vi "Index Event in Device List.vi"(8 "Error In":errorcluster, 11 "Device List State":T1) -> (0 "Error Out":errorcluster, 3 "Device List State out":T1, 4 "New Index":u32)   [LabVIEW 2015]
uses:
  Device List State.ctl
  Device/Device.lvclass
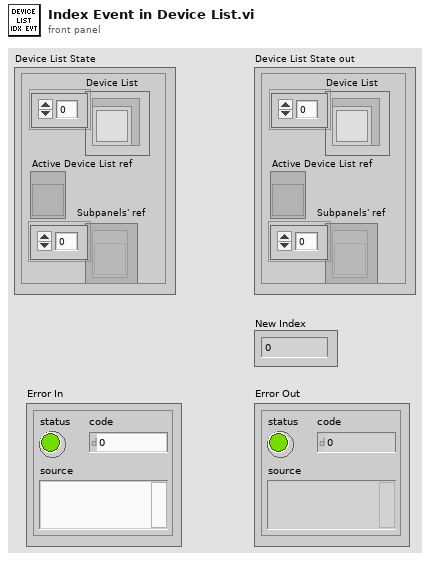
[diagram p1: front panel]
types:
  T1 = typedef "Device List State.ctl" = cluster{"Device List":refnum<class "Device.lvclass">[], "Active Device List ref":refnum<vi>, "Subpanels' ref":refnum<vi>[]}
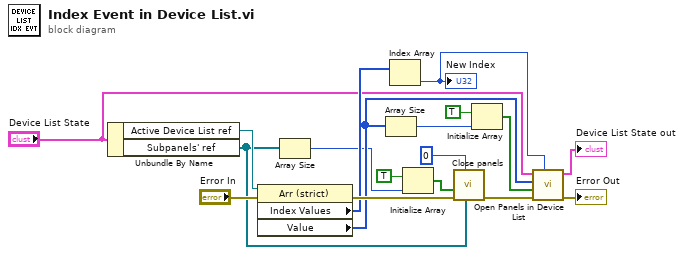
[diagram p0: block diagram]
diagram:
  n1 = Unbundle By Name("Device List State") -> ("Active Device List ref"=w3:refnum<vi>, "Subpanels' ref"=w1:refnum<vi>[])
  n2 = property class="Arr (strict)"(reference=w3, error in="Error In") -> (error out=w17:errorcluster, "Index Values"=w15:u32[], "Value"=w16:u16[])  [unwired: 1 out]
  n3 = Array Size(array=w1) -> (size(s)=w8:i32)
  n4 = Array Size(array=w16) -> (size(s)=w12:i32)
  n5 = Index Array(array=w15) -> (element=w14:u32)  [unwired: 1 in]
  "New Index" <- w14
  n6 = Initialize Array(TRUE, w8) -> (w5:bool[])
  n7 = call "Close panels.vi"("Subpanels' ref"=w1, "Index Value"=u32 0, "error in (no error)"=w17, "Subpanels to close"=w5) -> ("error out"=w10:errorcluster)  [unwired: 7 in]
  n8 = Initialize Array(TRUE, w12) -> (w6:bool[])
  n9 = call "Open Panels in Device List.vi"("Index Value"=w14, "error in (no error)"=w10, "Subpanels to open"=w6, "Active List"=w16, "Device List State"="Device List State") -> ("error out"=→"Error Out":errorcluster, "Device List State out"=→"Device List State out":T1)  [unwired: 5 in]
